vi "Teleop.vi"(0 "Call Context":T10) -> (6 "SubState 3":T1, 8 "SubState 4":T1, 9 "SubState 5":T9, 11 "Loop 3 Data":T5, 13 "Loop 4 Data":T4, 14 "SubState 0":T1=enum."driver control", 15 "Loop 1 Data":T7, 16 "Loop 0 Data":T8, 17 "SubState 1":T1, 18 "Loop 2 Data":T6, 19 "SubState 2":T1)   [LabVIEW 2013]
uses:
  typedefs/subStates.ctl
  <vilib>/Rock Robotics/WPI/DriverStation/WPI_DriverStationDerivedRobotMode.ctl
  typedefs/singleUseSubstate.ctl
  typedefs/Loop Datatypes/Loop 0 Datatype.ctl
  typedefs/Loop Datatypes/Loop 1 Datatype.ctl
  typedefs/Loop Datatypes/Loop 2 Datatype.ctl
  typedefs/Loop Datatypes/Loop 3 Datatype.ctl
  typedefs/Loop Datatypes/Loop 4 Datatype.ctl
  <vilib>/Rock Robotics/WPI/Joystick/WPI_JoystickDevRef.ctl
  <vilib>/Rock Robotics/WPI/Joystick/WPI_JoystickDeviceEnum.ctl
  typedefs/fg_typedef.ctl
  typedefs/vision enable.ctl
  <vilib>/Rock Robotics/WPI/Joystick/WPI_JoystickGetSetRefNum.vi
panel:
  out "prev lock state":T1
  out "JS3":T2
  out "Drive to DC":bool
  out "JS1":T2
  out "JS2":T2
  out "Exit Value":i32=-1
  # "Loop Data and Substates"
  # "Lock Loop"
  # "Drive Loop"
  # "Shooter Pneumatics Loop"
  # "Pickup/Passing Belts Loop"
  # "Pickup Arm Loop"
  # "Shifter Loop"
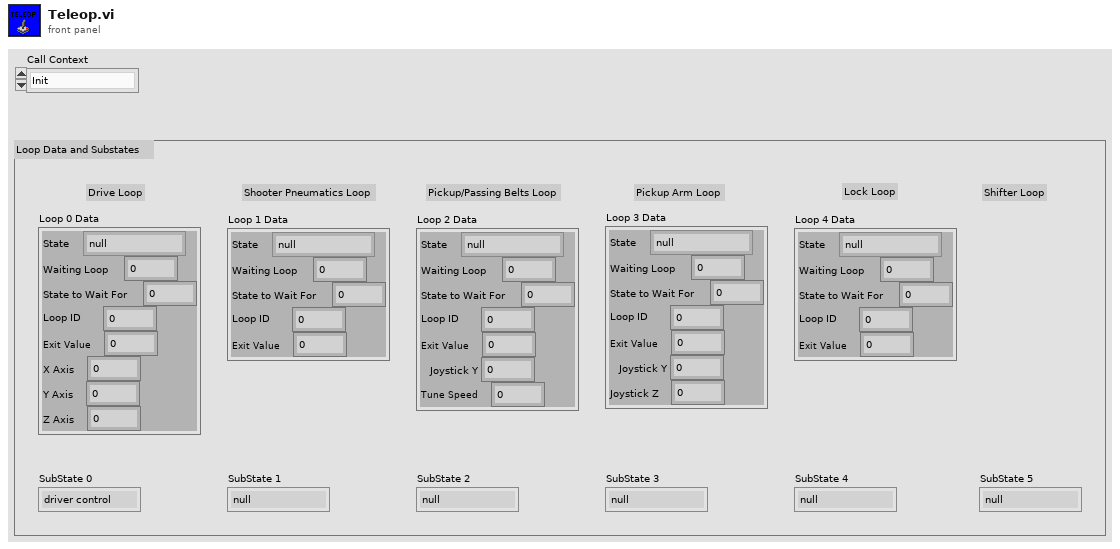
[diagram p1: front panel]
types:
  T1 = typedef "subStates.ctl" = enum16{"null", "wait", "driver control", "auto", "manual override", "hold position", "rotate", "pickup", "pass", "load", "goto shoot", "shoot", "end"}
  T2 = typedef "WPI_JoystickDevRef.ctl" = cluster{"Device":T3}
  T3 = typedef "WPI_JoystickDeviceEnum.ctl" = enum16{"USB 1", "USB 2", "USB 3", "USB 4", "Kinect 1", "Kinect 2"}
  T4 = typedef "Loop 4 Datatype.ctl" = cluster{"State":T1, "Waiting Loop":i32, "State to Wait For":i32, "Loop ID":i32, "Exit Value":i32}
  T5 = typedef "Loop 3 Datatype.ctl" = cluster{"State":T1, "Waiting Loop":i32, "State to Wait For":i32, "Loop ID":i32, "Exit Value":i32, "Joystick Y":dbl, "Joystick Z":dbl}
  T6 = typedef "Loop 2 Datatype.ctl" = cluster{"State":T1, "Waiting Loop":i32, "State to Wait For":i32, "Loop ID":i32, "Exit Value":i32, "Joystick Y":dbl, "Tune Speed":dbl}
  T7 = typedef "Loop 1 Datatype.ctl" = cluster{"State":T1, "Waiting Loop":i32, "State to Wait For":i32, "Loop ID":i32, "Exit Value":i32}
  T8 = typedef "Loop 0 Datatype.ctl" = cluster{"State":T1, "Waiting Loop":i32, "State to Wait For":i32, "Loop ID":i32, "Exit Value":i32, "X Axis":dbl, "Y Axis":dbl, "Z Axis":dbl}
  T9 = typedef "singleUseSubstate.ctl" = enum16{"null", "wait", "shift high", "shift low"}
  T10 = typedef "WPI_DriverStationDerivedRobotMode.ctl" = enum16{"Init", "Execute", "Stop"}
  T11 = cluster{"axis 1 (x)":dbl, "axis 2 (y)":dbl, "axis 3 (throttle)":dbl, "axis 4":dbl, "axis 5":dbl, "axis 6":dbl}
  T12 = typedef "WPI_EncoderDevRef.ctl" = cluster{"DevStatus":errorcluster, "EncoderIndex":T13, "CounterIndex":T14, "DistancePerCount":dbl, "Decoding Type":T15}
  T13 = typedef "FPGA_EncoderIdx.ctl" = enum8{"Enc 0", "Enc 1", "Enc 2", "Enc 3", "Invalid"}
  T14 = typedef "FPGA_CounterCtrSystemIndex.ctl" = enum8{"Ctr 0", "Ctr 1", "Ctr 2", "Ctr 3", "Ctr 4", "Ctr 5", "Ctr 6", "Ctr 7", "Invalid"}
  T15 = typedef "WPI_EncoderType.ctl" = enum16{"1x", "2x", "4x"}
  T16 = typedef "vision enable.ctl" = enum16{"Enable", "Disable", "Stop"}
  T17 = typedef "fg_typedef.ctl" = enum16{"Get", "Set"}
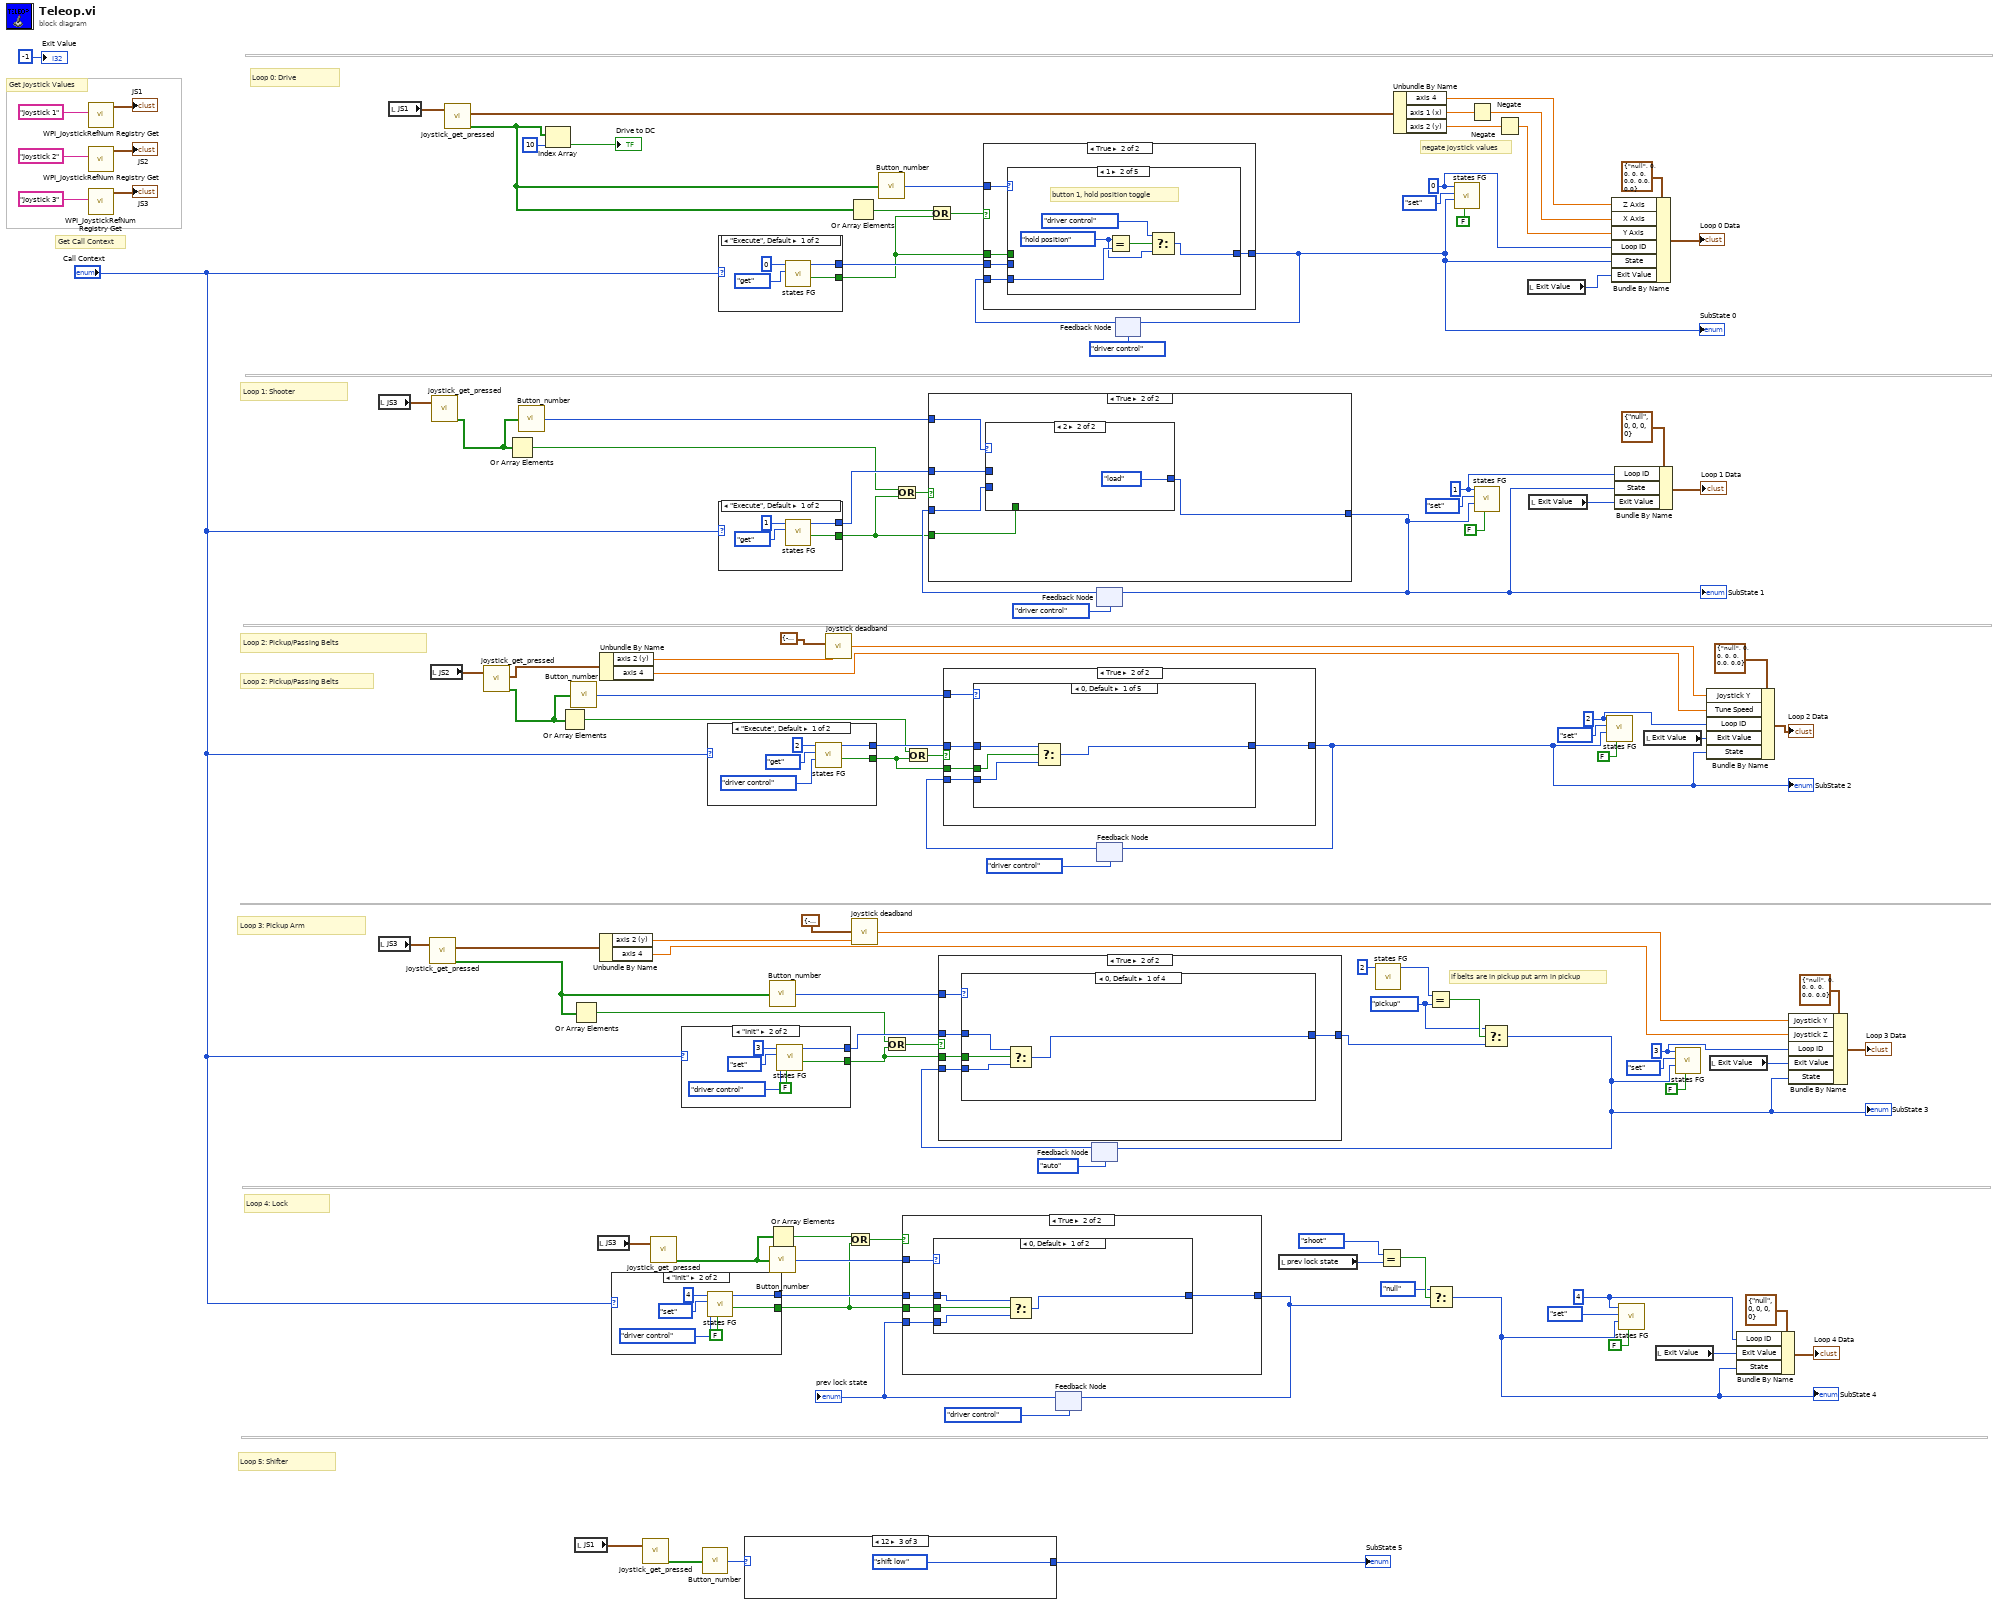
[diagram p0: block diagram]
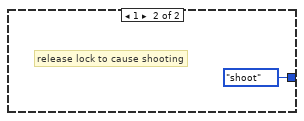
[diagram p3: hidden frame]
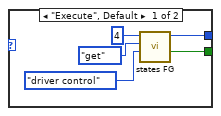
[diagram p4: hidden frame]
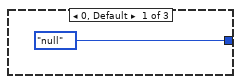
[diagram p5: hidden frame]
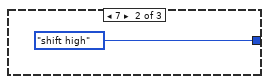
[diagram p6: hidden frame]
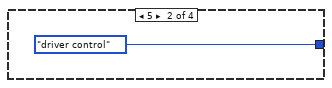
[diagram p8: hidden frame]
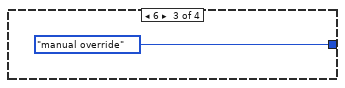
[diagram p9: hidden frame]
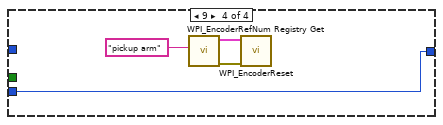
[diagram p10: hidden frame]
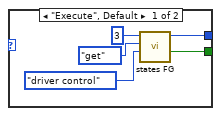
[diagram p11: hidden frame]
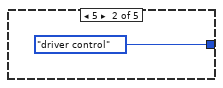
[diagram p13: hidden frame]
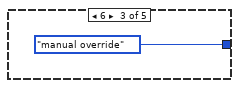
[diagram p14: hidden frame]
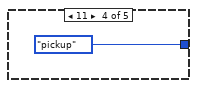
[diagram p15: hidden frame]
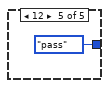
[diagram p16: hidden frame]
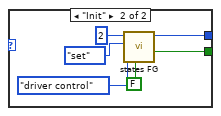
[diagram p17: hidden frame]
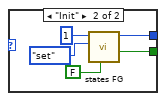
[diagram p18: hidden frame]
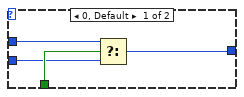
[diagram p20: hidden frame]
diagram:
  w7 = subStates."pickup" ("y")
  w26 = 4 ("Loop ID")
  w92 = 3 ("Loop ID")
  w93 = 2 ("Loop ID")
  w102 = 1 ("Loop ID")
  w104 = 0 ("Loop ID")
  # "if belts are in pickup put arm in pickup"
  # "Loop 2: Pickup/Passing Belts"
  # "negate joystick values"
  # "Get Call Context"
  # "Get Joystick Values"
  # "Loop 4: Lock"
  # "Loop 3: Pickup Arm"
  # "Loop 5: Shifter"
  # "Loop 2: Pickup/Passing Belts"
  # "Loop 1: Shooter"
  # "Loop 0: Drive"
  n1 = call <vilib>:"WPI_JoystickRefNum Registry Get.vi"("refnum name"="Joystick 1") -> ("JoystickDevRef"=→"JS1":T2)  [unwired: 9 in, 1 out]
  n2 = call <vilib>:"WPI_JoystickRefNum Registry Get.vi"("refnum name"="Joystick 2") -> ("JoystickDevRef"=→"JS2":T2)  [unwired: 9 in, 1 out]
  n3 = call <vilib>:"WPI_JoystickRefNum Registry Get.vi"("refnum name"="Joystick 3") -> ("JoystickDevRef"=→"JS3":T2)  [unwired: 9 in, 1 out]
  n4 = local read "JS3"() -> (w69:T2)
  n5 = local read "JS3"() -> (w54:T2)
  n6 = local read "JS1"() -> (w70:T2)
  n7 = call "joystick_get_pressed.vi"("JoystickDevRef 2"=w54) -> ("Axes"=w58:T11, "Buttons Pressed?"=w35:bool[])  [unwired: 1 in, 2 out]
  n8 = local read "JS2"() -> (w42:T2)
  n9 = call "joystick_get_pressed.vi"("JoystickDevRef 2"=w69) -> ("Buttons Pressed?"=w37:bool[])  [unwired: 1 in, 3 out]
  n10 = call "joystick_get_pressed.vi"("JoystickDevRef 2"=w70) -> ("Axes"=w74:T11, "Buttons Pressed?"=w50:bool[])  [unwired: 1 in, 2 out]
  n11 = call "joystick_get_pressed.vi"("JoystickDevRef 2"=w42) -> ("Axes"=w23:T11, "Buttons Pressed?"=w24:bool[])  [unwired: 1 in, 2 out]
  n12 = Or Array Elements(Boolean array=w37) -> (logical OR=w61:bool)
  n13 = call "Button_number.vi"("Button Array"=w37) -> ("Button Pressed"=w63:i32)
  n14 = Index Array(array=w50, index=10) -> (element=→"Drive to DC":bool)
  n15 = Or Array Elements(Boolean array=w24) -> (logical OR=w41:bool)
  n16 = call "Button_number.vi"("Button Array"=w24) -> ("Button Pressed"=w40:i32)
  n17 = Or Array Elements(Boolean array=w35) -> (logical OR=w57:bool)
  n18 = local read "JS1"() -> (w45:T2)
  n19 = local read "JS3"() -> (w18:T2)
  n20 = Unbundle By Name(w58) -> ("axis 2 (y)"=w53:dbl, "axis 4"=w19:dbl)
  n21 = Unbundle By Name(w23) -> ("axis 2 (y)"=w34:dbl, "axis 4"=w21:dbl)
  n22 = case shown="\"Init\"" "Call Context" {
    tunnel: [w123 w129] -> w13
    tunnel: [w121 w126] -> w28
    frame "Execute", Default {
      n23 = call "states FG.vi"("subState in"=subStates."driver control", "menu (get)"=enum16{"set", "get"}."get", "Loop ID"=4) -> ("exit out"=w123:bool, "subState out"=w121:T1)  [unwired: 5 in, 2 out]
    }
    frame "Init" {
      n24 = call "states FG.vi"("exit in"=FALSE, "subState in"=subStates."driver control", "menu (get)"=enum16{"set", "get"}."set", "Loop ID"=4) -> ("exit out"=w129:bool, "subState out"=w126:T1)  [unwired: 4 in, 2 out]
    }
  }
  n25 = call "joystick_get_pressed.vi"("JoystickDevRef 2"=w45) -> ("Buttons Pressed?"=w47:bool[])  [unwired: 1 in, 3 out]
  n26 = call "joystick_get_pressed.vi"("JoystickDevRef 2"=w18) -> ("Buttons Pressed?"=w17:bool[])  [unwired: 1 in, 3 out]
  n27 = case shown="\"Init\"" "Call Context" {
    tunnel: [w134 w140] -> w55
    tunnel: [w132 w137] -> w90
    frame "Execute", Default {
      n28 = call "states FG.vi"("subState in"=subStates."driver control", "menu (get)"=enum16{"set", "get"}."get", "Loop ID"=3) -> ("exit out"=w134:bool, "subState out"=w132:T1)  [unwired: 5 in, 2 out]
    }
    frame "Init" {
      n29 = call "states FG.vi"("exit in"=FALSE, "subState in"=subStates."driver control", "menu (get)"=enum16{"set", "get"}."set", "Loop ID"=3) -> ("exit out"=w140:bool, "subState out"=w137:T1)  [unwired: 4 in, 2 out]
    }
  }
  n30 = call "Button_number.vi"("Button Array"=w47) -> ("Button Pressed"=w46:i32)
  n31 = case shown="\"Execute\", Default" "Call Context" {
    tunnel: [w145 w151] -> w60
    tunnel: [w143 w148] -> w109
    frame "Execute", Default {
      n32 = call "states FG.vi"("subState in"=subStates."driver control", "menu (get)"=enum16{"set", "get"}."get", "Loop ID"=2) -> ("exit out"=w145:bool, "subState out"=w143:T1)  [unwired: 5 in, 2 out]
    }
    frame "Init" {
      n33 = call "states FG.vi"("exit in"=FALSE, "subState in"=subStates."driver control", "menu (get)"=enum16{"set", "get"}."set", "Loop ID"=2) -> ("exit out"=w151:bool, "subState out"=w148:T1)  [unwired: 4 in, 2 out]
    }
  }
  n34 = case shown="\"Execute\", Default" "Call Context" {
    tunnel: [w155 w160] -> w67
    tunnel: [w154 w158] -> w107
    frame "Execute", Default {
      n35 = call "states FG.vi"("menu (get)"=enum16{"set", "get"}."get", "Loop ID"=0) -> ("exit out"=w155:bool, "subState out"=w154:T1)  [unwired: 6 in, 2 out]
    }
    frame "Init" {
      n36 = call "states FG.vi"("exit in"=FALSE, "menu (get)"=enum16{"set", "get"}."set", "Loop ID"=0) -> ("exit out"=w160:bool, "subState out"=w158:T1)  [unwired: 5 in, 2 out]
    }
  }
  n37 = case shown="\"Execute\", Default" "Call Context" {
    tunnel: [w164 w169] -> w64
    tunnel: [w163 w167] -> w106
    frame "Execute", Default {
      n38 = call "states FG.vi"("menu (get)"=enum16{"set", "get"}."get", "Loop ID"=1) -> ("exit out"=w164:bool, "subState out"=w163:T1)  [unwired: 6 in, 2 out]
    }
    frame "Init" {
      n39 = call "states FG.vi"("exit in"=FALSE, "menu (get)"=enum16{"set", "get"}."set", "Loop ID"=1) -> ("exit out"=w169:bool, "subState out"=w167:T1)  [unwired: 5 in, 2 out]
    }
  }
  n40 = case shown="12" w46 {
    tunnel: [singleUseSubstate."null" ("Enum") singleUseSubstate."shift high" ("Enum") singleUseSubstate."shift low" ("Enum")] -> w82
    frame 0, Default {
    }
    frame 7 {
    }
    frame 12 {
    }
  }
  "SubState 5" <- w82
  n41 = call "Button_number.vi"("Button Array"=w35) -> ("Button Pressed"=w56:i32)
  n42 = call "Button_number.vi"("Button Array"=w17) -> ("Button Pressed"=w14:i32)
  n43 = Or Array Elements(Boolean array=w17) -> (logical OR=w16:bool)
  n44 = call "joystick deadband.vi"("Joystick In"=w34, "Deadband Range"=cluster{"Deadband Min":dbl, "Deadband Max":dbl} {"Deadband Min"=-0.05, "Deadband Max"=0.05}) -> ("Joystick Out"=w22:dbl)  [unwired: 4 in]
  n45 = Or(x=w16, y=w13) -> (x .or. y?=w15:bool)
  n46 = Or Array Elements(Boolean array=w50) -> (logical OR=w68:bool)
  n47 = call "joystick deadband.vi"("Joystick In"=w53, "Deadband Range"=cluster{"Deadband Min":dbl, "Deadband Max":dbl} {"Deadband Min"=-0.05, "Deadband Max"=0.05}) -> ("Joystick Out"=w20:dbl)  [unwired: 4 in]
  n48 = call "Button_number.vi"("Button Array"=w50) -> ("Button Pressed"=w73:i32)
  n49 = Or(x=w57, y=w55) -> (x .or. y?=w59:bool)
  n50 = Or(x=w61, y=w64) -> (x .or. y?=w65:bool)
  n51 = Or(x=w41, y=w60) -> (x .or. y?=w62:bool)
  n52 = Or(x=w68, y=w67) -> (x .or. y?=w66:bool)
  n53 = feedback #1(subStates."driver control" ("Drive SubState")) -> (w31:T1)
  "prev lock state" <- w31
  n54 = case shown="True" w15 {
    tunnel: w31 -> [w175 w177]
    tunnel: [w175 w176] -> w3
    tunnel: w28 -> [_ w179]
    tunnel: w14 -> [_ w180]
    tunnel: w13 -> [_ w178]
    frame False {
      # "*yawn* nothing to do...wire through the previous state"
    }
    frame True {
      n55 = case shown="0, Default" w180 {
        tunnel: w179 -> [w183 _]
        tunnel: w178 -> [w184 _]
        tunnel: w177 -> [w182 _]
        tunnel: [w181 subStates."shoot" ("Drive SubState")] -> w176
        frame 0, Default {
          n56 = Select(t=w183, s=w184, f=w182) -> (s? t:f=w181:T1)
        }
        frame 1 {
          # "release lock to cause shooting"
        }
      }
    }
  }
  n57 = feedback-in #1(w3) -> ()
  n58 = feedback #2(subStates."auto" ("Drive SubState")) -> (w87:T1)
  n59 = case shown="True" w59 {
    tunnel: w87 -> [w186 w187]
    tunnel: [w186 w188] -> w10
    tunnel: w90 -> [_ w189]
    tunnel: w56 -> [_ w191]
    tunnel: w55 -> [_ w190]
    frame False {
      # "boring drivers, not pressing anything...wire through the previous state"
    }
    frame True {
      n60 = case shown="0, Default" w191 {
        tunnel: w190 -> [w195 _ _ _]
        tunnel: w187 -> [w194 _ _ w201]
        tunnel: w189 -> [w193 _ _ _]
        tunnel: [w192 subStates."driver control" ("Drive SubState") subStates."manual override" ("Drive SubState") w201] -> w188
        frame 0, Default {
          n61 = Select(t=w193, s=w195, f=w194) -> (s? t:f=w192:T1)
        }
        frame 5 {
        }
        frame 6 {
        }
        frame 9 {
          n62 = call <vilib>:"WPI_EncoderRefNum Registry Get.vi"("refnum name"="pickup arm") -> ("error out"=w199:errorcluster, "EncoderDevRef"=w198:T12)  [unwired: 9 in]
          n63 = call <vilib>:"WPI_EncoderReset.vi"("error in (no error)"=w199, "EncoderDevRef"=w198) -> ()  [unwired: 8 in, 2 out]
        }
      }
    }
  }
  n64 = feedback #3(subStates."driver control" ("Drive SubState")) -> (w108:T1)
  n65 = case shown="True" w65 {
    tunnel: w108 -> [w202 w206]
    tunnel: [w202 w203] -> w75
    tunnel: w106 -> [_ w207]
    tunnel: w63 -> [_ w205]
    tunnel: w64 -> [_ w204]
    frame False {
      # "nothing pressed here, move along (wire through the previous state)"
    }
    frame True {
      n66 = case shown="2" w205 {
        tunnel: w207 -> [w210 _]
        tunnel: w206 -> [w209 _]
        tunnel: [w208 subStates."load" ("Drive SubState")] -> w203
        tunnel: w204 -> [w211 _]
        frame 0, Default {
          n67 = Select(t=w210, s=w211, f=w209) -> (s? t:f=w208:T1)
        }
        frame 2 {
        }
      }
    }
  }
  "SubState 1" <- w75
  n68 = feedback-in #3(w75) -> ()
  n69 = feedback #4(subStates."driver control" ("Drive SubState")) -> (w112:T1)
  n70 = case shown="True" w62 {
    tunnel: w112 -> [w213 w215]
    tunnel: [w213 w214] -> w33
    tunnel: w109 -> [_ w216]
    tunnel: w40 -> [_ w218]
    tunnel: w60 -> [_ w217]
    frame False {
      # "nothing pressed here, move along obviously and wire through the previous state"
    }
    frame True {
      n71 = case shown="0, Default" w218 {
        tunnel: w217 -> [w222 _ _ _ _]
        tunnel: w216 -> [w221 _ _ _ _]
        tunnel: w215 -> [w220 _ _ _ _]
        tunnel: [w219 subStates."driver control" ("Drive SubState") subStates."manual override" ("Drive SubState") subStates."pickup" ("Drive SubState") subStates."pass" ("Drive SubState")] -> w214
        frame 0, Default {
          n72 = Select(t=w221, s=w222, f=w220) -> (s? t:f=w219:T1)
        }
        frame 5 {
        }
        frame 6 {
        }
        frame 11 {
        }
        frame 12 {
        }
      }
    }
  }
  "SubState 2" <- w33
  n73 = feedback-in #4(w33) -> ()
  n74 = feedback #5(subStates."driver control" ("Drive SubState")) -> (w114:T1)
  n75 = case shown="True" w66 {
    tunnel: w114 -> [w227 w229]
    tunnel: [w227 w228] -> w44
    tunnel: w107 -> [_ w230]
    tunnel: w73 -> [_ w232]
    tunnel: w67 -> [_ w231]
    frame False {
      # "keep current state, no change necessary"
    }
    frame True {
      n76 = case shown="1" w232 {
        tunnel: w231 -> [w236 _ _ _ _]
        tunnel: w230 -> [w235 _ _ _ _]
        tunnel: w229 -> [w234 w241 w242 _ _]
        tunnel: [w233 w237 w242 subStates."goto shoot" ("Drive SubState") subStates."driver control" ("Drive SubState")] -> w228
        frame 0, Default {
          n77 = Select(t=w235, s=w236, f=w234) -> (s? t:f=w233:T1)
        }
        frame 1 {
          w238 = subStates."hold position" ("x")
          # "button 1, hold position toggle"
          n78 = Equal?(x=w238, y=w241) -> (x = y?=w240:bool)
          n79 = Select(t=subStates."driver control" ("Drive SubState"), s=w240, f=w238) -> (s? t:f=w237:T1)
        }
        frame 8 {
          w245 = vision_enable."Enable" ("y")
          # "toggle vision"
          n80 = call "vision_fg.vi"("Menu"=fg_typedef."Get") -> ("State Out"=w247:T16)  [unwired: 2 in, 1 out]
          n81 = Equal?(x=w247, y=w245) -> (x = y?=w246:bool)
          n82 = Select(t=vision_enable."Disable" ("y"), s=w246, f=w245) -> (s? t:f=w243:T16)
          n83 = call "vision_fg.vi"("Action"=w243, "Menu"=fg_typedef."Set") -> ()  [unwired: 1 in, 2 out]
        }
        frame 9 {
          # "go to shoot location"
          n84 = call "vision_fg.vi"("Action"=vision_enable."Enable", "Menu"=fg_typedef."Set") -> ()  [unwired: 1 in, 2 out]
        }
        frame 11 {
          # "put robot drive in driver control"
          n85 = call "vision_fg.vi"("Action"=vision_enable."Disable", "Menu"=fg_typedef."Set") -> ()  [unwired: 1 in, 2 out]
        }
      }
    }
  }
  "SubState 0" <- w44
  n86 = feedback-in #5(w44) -> ()
  n87 = local read "prev lock state"() -> (w6:T1)
  n88 = call "states FG.vi"("Loop ID"=2) -> ("subState out"=w11:T1)  [unwired: 7 in, 3 out]
  n89 = Equal?(x=subStates."shoot", y=w6) -> (x = y?=w4:bool)
  n90 = Unbundle By Name(w74) -> ("axis 4"=w51:dbl, "axis 1 (x)"=w79:dbl, "axis 2 (y)"=w78:dbl)
  n91 = Equal?(x=w11, y=w7) -> (x = y?=w8:bool)
  n92 = Select(t=subStates."null", s=w4, f=w3) -> (s? t:f=w2:T1)
  "SubState 4" <- w2
  n93 = call "states FG.vi"("exit in"=FALSE, "subState in"=w44, "menu (get)"=enum16{"set", "get"}."set", "Loop ID"=w104) -> ()  [unwired: 4 in, 4 out]
  n94 = Negate(x=w79) -> (-x=w77:dbl)
  n95 = call "states FG.vi"("exit in"=FALSE, "subState in"=w75, "menu (get)"=enum16{"set", "get"}."set", "Loop ID"=w102) -> ()  [unwired: 4 in, 4 out]
  n96 = Select(t=w7, s=w8, f=w10) -> (s? t:f=w9:T1)
  "SubState 3" <- w9
  n97 = feedback-in #2(w9) -> ()
  n98 = Negate(x=w78) -> (-x=w76:dbl)
  n99 = local read "Exit Value"() -> (w100:i32)
  n100 = local read "Exit Value"() -> (w99:i32)
  n101 = call "states FG.vi"("exit in"=FALSE, "subState in"=w33, "menu (get)"=enum16{"set", "get"}."set", "Loop ID"=w93) -> ()  [unwired: 4 in, 4 out]
  n102 = Bundle By Name(cluster=T8 {"State"=enum."null", "Waiting Loop"=0, "State to Wait For"=0, "Loop ID"=0, "Exit Value"=0, "X Axis"=0.0, "Y Axis"=0.0, "Z Axis"=0.0} ("Cluster"), "Z Axis"=w51, "X Axis"=w77, "Y Axis"=w76, "Loop ID"=w104, "State"=w44, "Exit Value"=w100) -> (→"Loop 0 Data":T8)
  n103 = Bundle By Name(cluster=T7 {"State"=enum."null", "Waiting Loop"=0, "State to Wait For"=0, "Loop ID"=0, "Exit Value"=0} ("Cluster"), "Loop ID"=w102, "State"=w75, "Exit Value"=w99) -> (→"Loop 1 Data":T7)
  n104 = call "states FG.vi"("exit in"=FALSE, "subState in"=w2, "menu (get)"=enum16{"set", "get"}."set", "Loop ID"=w26) -> ()  [unwired: 4 in, 4 out]
  n105 = local read "Exit Value"() -> (w94:i32)
  n106 = local read "Exit Value"() -> (w27:i32)
  n107 = call "states FG.vi"("exit in"=FALSE, "subState in"=w9, "menu (get)"=enum16{"set", "get"}."set", "Loop ID"=w92) -> ()  [unwired: 4 in, 4 out]
  n108 = Bundle By Name(cluster=T6 {"State"=enum."null", "Waiting Loop"=0, "State to Wait For"=0, "Loop ID"=0, "Exit Value"=0, "Joystick Y"=0.0, "Tune Speed"=0.0} ("Loop 2 Data"), "Joystick Y"=w22, "Tune Speed"=w21, "Loop ID"=w93, "Exit Value"=w94, "State"=w33) -> (→"Loop 2 Data":T6)
  n109 = local read "Exit Value"() -> (w91:i32)
  n110 = Bundle By Name(cluster=T4 {"State"=enum."null", "Waiting Loop"=0, "State to Wait For"=0, "Loop ID"=0, "Exit Value"=0} ("Loop 4 Data"), "Loop ID"=w26, "Exit Value"=w27, "State"=w2) -> (→"Loop 4 Data":T4)
  n111 = Bundle By Name(cluster=T5 {"State"=enum."null", "Waiting Loop"=0, "State to Wait For"=0, "Loop ID"=0, "Exit Value"=0, "Joystick Y"=0.0, "Joystick Z"=0.0} ("Loop 3 Data"), "Joystick Y"=w20, "Joystick Z"=w19, "Loop ID"=w92, "Exit Value"=w91, "State"=w9) -> (→"Loop 3 Data":T5)
  "Exit Value" <- -1 ("Exit Value")
